vi "zad1.vi"() -> ()   [LabVIEW 2018]
panel:
  out "Waveform Chart":i32(graph)
  in  "stop":bool
  out "standard output":string
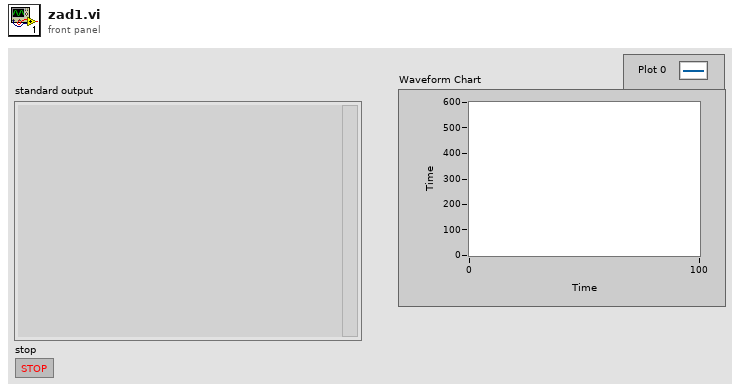
[diagram p1: front panel]
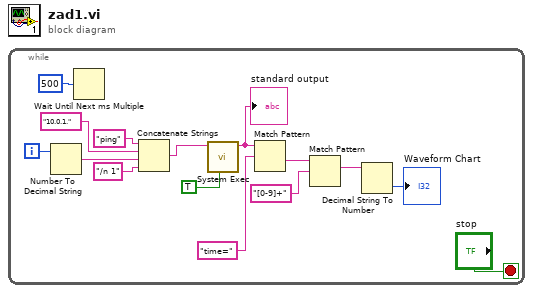
[diagram p0: block diagram]
diagram:
  n1 = while {
    i -> [w6]
    stop <- "stop" stop-if-true
    n2 = Number To Decimal String(number=w6) -> (decimal integer string=w3:string)  [unwired: 1 in]
    n3 = Wait Until Next ms Multiple(millisecond multiple=u32 500) -> ()  [unwired: 1 out]
    n4 = Concatenate Strings("ping" ("command line"), "10.0.1.", w3, "/n 1") -> (w1:string)
    n5 = call <vilib>:"System Exec.vi"("run minimized? (F)"=TRUE, "command line"=w1) -> ("standard output"=w12:string)  [unwired: 6 in, 3 out]
    "standard output" <- w12
    n6 = Match Pattern(string=w12, regular expression="time=" ("search string")) -> (after substring=w10:string)  [unwired: 1 in, 3 out]
    n7 = Match Pattern(string=w10, regular expression="[0-9]+") -> (match substring=w8:string)  [unwired: 1 in, 3 out]
    n8 = Decimal String To Number(string=w8) -> (number=→"Waveform Chart":i32)  [unwired: 2 in, 1 out]
  }
